vi "Example Find Borders - PositionReached Callback.vi"(4 "PositionReached":refnum<user-event>, 5 "Event Data":cluster{"sender":refnum<k24>, "x":i16, "y":i16}, 6 "Control Ref":refnum<k24>, 7 "Event Common Data":T1) -> ()   [LabVIEW 2013]
uses:
  C:/tf/play/labview/Tinkerforge.dll
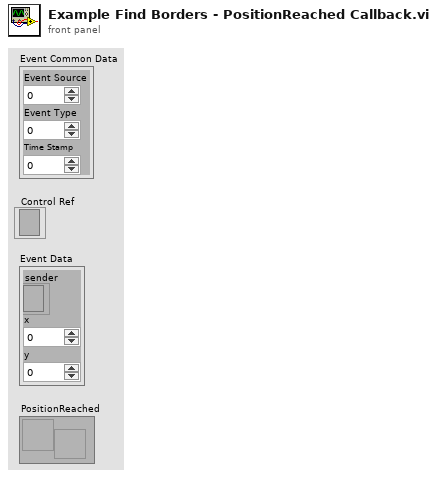
[diagram p1: front panel]
types:
  T1 = cluster{"Event Source":i32, "Event Type":u32, "Time Stamp":u32}
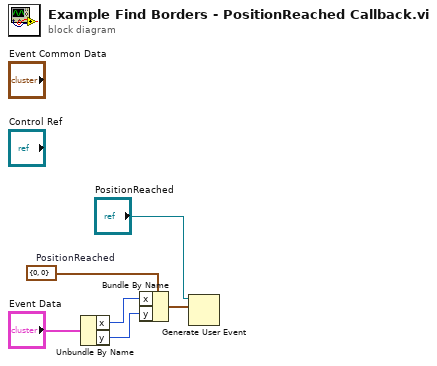
[diagram p0: block diagram]
diagram:
  w5 = cluster{"x":i16, "y":i16} {"x"=0, "y"=0}  # PositionReached
  n1 = Unbundle By Name("Event Data") -> ("x"=w3:i16, "y"=w2:i16)
  n2 = Bundle By Name(cluster=w5, "x"=w3, "y"=w2) -> (w6:cluster{"x":i16, "y":i16})
  n3 = Generate User Event(user event="PositionReached", event data cluster=w6) -> ()  [unwired: 2 in, 2 out]
